vi "PhotonPipelineResult_Equals.vi"(9 "Other PhotonPipelineResult_REF":T1, 11 "PhotonPipelineResult_REF":T1) -> (3 "Equal":bool)   [LabVIEW 2019, in "PhotonVisionLib.lvlib"]
doc: "Determines if two PipelineResults are equal.\n\nInputs:\n - PipelineResult -- PipelineResult cluster.\n - Other PipelineResult -- Other PipelineResult cluster.\n\nOutputs:\n - Equal -- Returns TRUE, if both pipeline results are equal.."
uses:
  PhotonVisionLib.lvlib
  TypeDef/TargetCornerType.ctl
  TypeDef/PhotonTrackedTargetType.ctl
  TypeDef/PhotonPipelineResultType.ctl
  <vilib>/Rock Robotics/WPI/ThirdParty/JAS_Junk/TrajLib/TypeDef/TRANSLATION3D.ctl
  <vilib>/Rock Robotics/WPI/ThirdParty/JAS_Junk/TrajLib/Trajectory_Library.lvlib
  <vilib>/Rock Robotics/WPI/ThirdParty/JAS_Junk/TrajLib/TypeDef/QUATERNION.ctl
  <vilib>/Rock Robotics/WPI/ThirdParty/JAS_Junk/TrajLib/TypeDef/ROTATION3D.ctl
  <vilib>/Rock Robotics/WPI/ThirdParty/JAS_Junk/TrajLib/TypeDef/TRANSFORM3D.ctl
  TypeDef/PhotonPNPResultType.ctl
  TypeDef/PhotonMultiTargetPNPResultType.ctl
  Ref/PhotonPipelineResult_REF.ctl
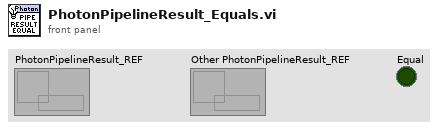
[diagram p1: front panel]
types:
  T1 = typedef "PhotonVisionLib.lvlib/PhotonPipelineResult_REF.ctl" = refnum<data-value>
  T2 = typedef "PhotonVisionLib.lvlib/PhotonTrackedTargetType.ctl" = cluster{"Yaw":dbl, "Pitch":dbl, "Area":dbl, "Skew":dbl, "MinAreaRectCorners":T3[], "BestCameraToTarget":T4, "FiiducialId":i32, "AltCameraToTarget":T4, "PoseAmbiguity":dbl, "DetectedCorners":T3[]}
  T3 = typedef "PhotonVisionLib.lvlib/TargetCornerType.ctl" = cluster{"X":dbl, "Y":dbl}
  T4 = typedef "Trajectory_Library.lvlib/TRANSFORM3D.ctl" = cluster{"TRANSLATION3D":T5, "ROTATION3D":T6, "XF":bool}
  T5 = typedef "Trajectory_Library.lvlib/TRANSLATION3D.ctl" = cluster{"X":dbl, "Y":dbl, "Z":dbl}
  T6 = typedef "Trajectory_Library.lvlib/ROTATION3D.ctl" = cluster{"Q_quaternion":T7}
  T7 = typedef "Trajectory_Library.lvlib/QUATERNION.ctl" = cluster{"R":dbl, "V":dbl[]}
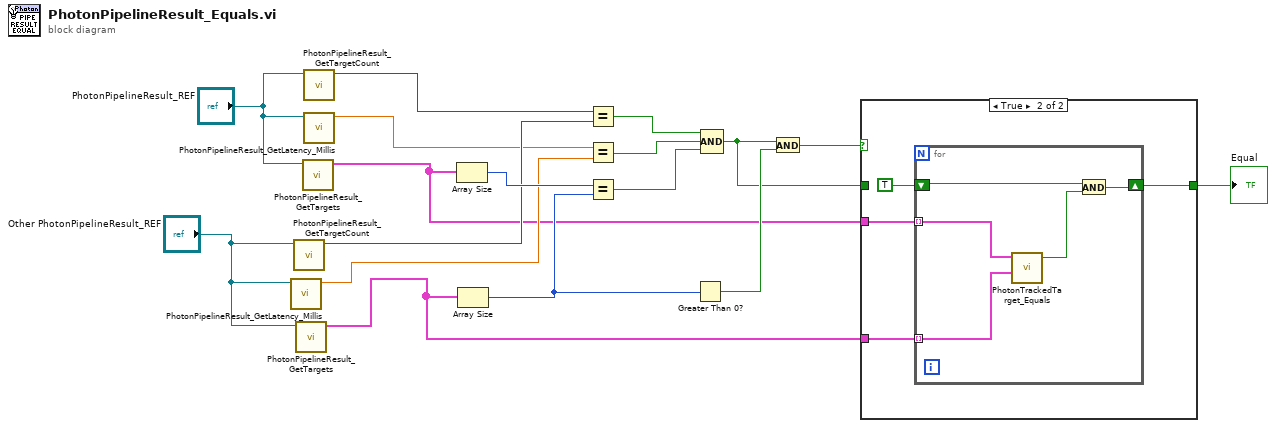
[diagram p0: block diagram]
diagram:
  n1 = call "PhotonPipelineResult_GetLatency_Millis.vi"("PhotonPipelineResult_REF"="Other PhotonPipelineResult_REF") -> ("Latency_MilliSec"=w5:dbl)  [unwired: 9 in, 1 out]
  n2 = call "PhotonPipelineResult_GetTargetCount.vi"("PhotonPipelineResult_REF"="Other PhotonPipelineResult_REF") -> ("TargetCount"=w6:i32)  [unwired: 10 in]
  n3 = call "PhotonPipelineResult_GetTargets.vi"("PhotonPipelineResult_REF"="Other PhotonPipelineResult_REF") -> ("Targets"=w4:T2[])  [unwired: 10 in]
  n4 = call "PhotonPipelineResult_GetTargets.vi"("PhotonPipelineResult_REF"="PhotonPipelineResult_REF") -> ("Targets"=w1:T2[])  [unwired: 10 in]
  n5 = call "PhotonPipelineResult_GetTargetCount.vi"("PhotonPipelineResult_REF"="PhotonPipelineResult_REF") -> ("TargetCount"=w3:i32)  [unwired: 10 in]
  n6 = call "PhotonPipelineResult_GetLatency_Millis.vi"("PhotonPipelineResult_REF"="PhotonPipelineResult_REF") -> ("Latency_MilliSec"=w2:dbl)  [unwired: 9 in, 1 out]
  n7 = Array Size(array=w1) -> (size(s)=w17:i32)
  n8 = Array Size(array=w4) -> (size(s)=w13:i32)
  n9 = Equal?(x=w3, y=w6) -> (x = y?=w16:bool)
  n10 = Equal?(x=w2, y=w5) -> (x = y?=w15:bool)
  n11 = Equal?(x=w17, y=w13) -> (x = y?=w14:bool)
  n12 = Greater Than 0?(x=w13) -> (x > 0?=w12:bool)
  n13 = Compound Arithmetic op=AND(w16, w15, w14) -> (w9:bool)
  n14 = And(x=w9, y=w12) -> (x .and. y?=w11:bool)
  n15 = case shown="True" w11 {
    tunnel: w1 -> [_ w22]
    tunnel: w4 -> [_ w21]
    tunnel: [w18 w19] -> w10
    tunnel: w9 -> [w18 _]
    frame False {
    }
    frame True {
      n16 = for {
        tunnel: w22 -> [w27] mode=indexing
        tunnel: w21 -> [w26] mode=indexing
        shift-right: [w25] -> w19
        shift-left: TRUE -> [w24]
        n17 = call "PhotonTrackedTarget_Equals.vi"("Other TrackedTarget"=w26, "TrackedTarget"=w27) -> ("Equals"=w23:bool)  [unwired: 9 in]
        n18 = And(x=w24, y=w23) -> (x .and. y?=w25:bool)
      }
    }
  }
  "Equal" <- w10
